vi "Reset Supply.vi"(8 "error in":errorcluster, 11 "IF_XX in":refnum<class "IF_XX.lvclass">) -> (0 "error out":errorcluster, 3 "IF_XX out":refnum<class "IF_XX.lvclass">)   [LabVIEW 2019, in "IF_XX.lvlib" / "IF_XX.lvclass"]
uses:
  Library/IF_XX.lvclass
  Library/IF_XX.lvclass/IF_XX.ctl
  builds/Instruments/PowerSupply.lvlibp/Library/PowerSupply.lvclass
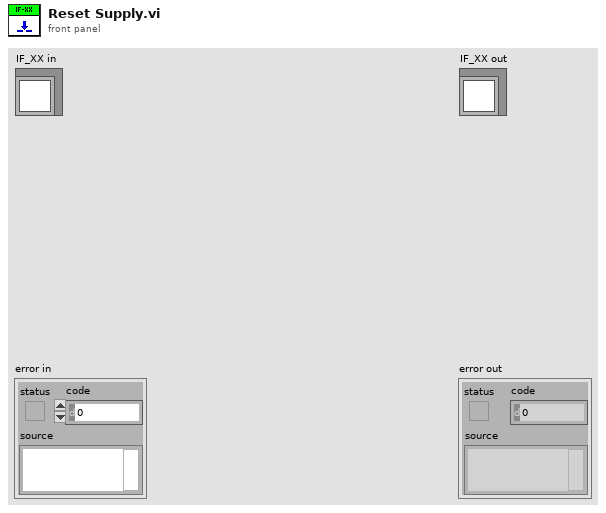
[diagram p1: front panel]
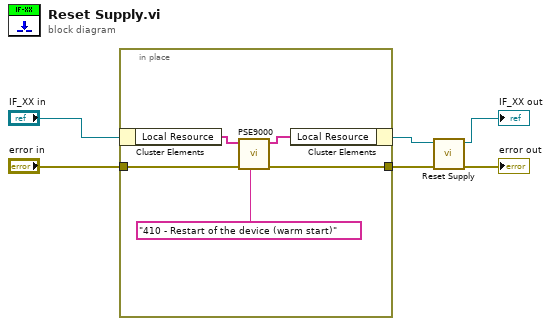
[diagram p0: block diagram]
diagram:
  n1 = in-place {
    in-place-border: "error in" -> [w9]
    in-place-border: [w8] -> w3
    n2 = in-place-cluster #1("IF_XX in") -> ("Local Resource"=w11:string[])
    n3 = call <instrlib>:"PSE9000.vi"("Command list"="410 - Restart of the device (warm start)", "Error in"=w9, "Device information in"=w11) -> ("Error out"=w8:errorcluster, "Device information out"=w10:string[])  [unwired: 3 in, 2 out]
    n4 = in-place-cluster #1("Local Resource"=w10) -> (w4:refnum<class "IF_XX.lvclass">)
  }
  n5 = call-parent "Reset Supply.vi"("error in"=w3, "PowerSupply in"=w4) -> ("error out"=→"error out":errorcluster, "PowerSupply out"=→"IF_XX out":refnum<class "IF_XX.lvclass">)  [unwired: 8 in]
